vi "ttl_high_low.vi"(4 "lines":tag="Dev1/port2/line7", 7 "Boolean":bool=TRUE) -> ()   [LabVIEW 2011]
uses:
  <vilib>/DAQmx/write.llb/DAQmx Write (Digital 1D Bool 1Chan 1Samp).vi
  <vilib>/DAQmx/create/channels.llb/DAQmx Create Channel (DO-Digital Output).vi
  <vilib>/DAQmx/miscellaneous.llb/DAQmx Fill In Error Info.vi
  Program Files/National Instruments/LabVIEW 2011/resource/objmgr/daqmx.rc
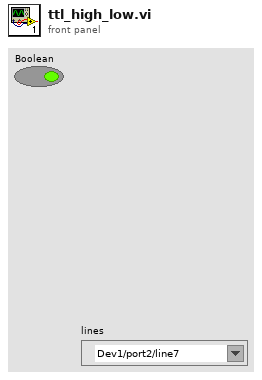
[diagram p1: front panel]
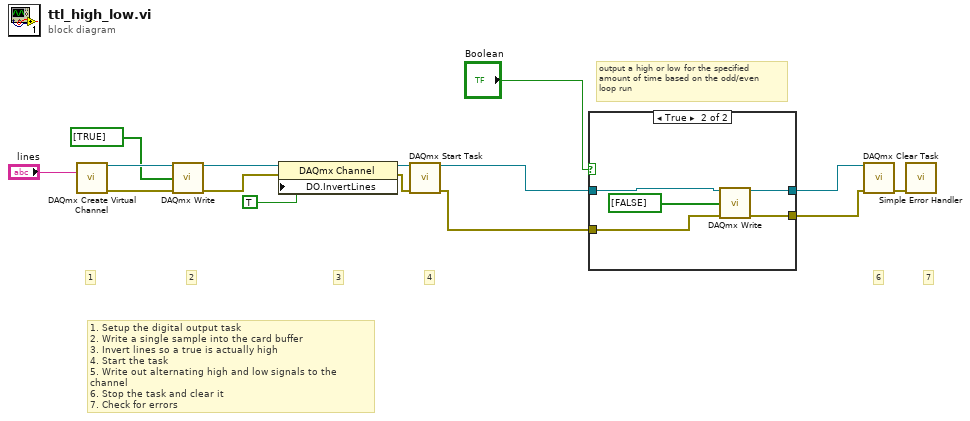
[diagram p0: block diagram]
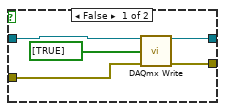
[diagram p2: hidden frame]
diagram:
  # "output a high or low for the specified\namount of time based on the odd/even\nloop run"
  # "1. Setup the digital output task\n2. Write a single sample into the card buffer\n3. Invert lines so a true is actually high\n4. Start the task\n5. Write out alternating high and low signals to the channel\n6. Stop the task and clear it\n7. Check for errors"
  # "7"
  # "6"
  # "4"
  # "3"
  # "2"
  # "1"
  n1 = call-poly <vilib>:"DAQmx Create Virtual Channel.vi"("lines"="lines") -> ("task out"=w15:refnum<k21>, "error out"=w14:errorcluster)  [unwired: 13 in]
  n2 = call-poly <vilib>:"DAQmx Write.vi"("task/channels in"=w15, "data"=bool[] [TRUE], "error in"=w14) -> ("task out"=w10:refnum<k21>, "error out"=w6:errorcluster)  [unwired: 10 in, 1 out]
  n3 = property class="DAQmx Channel"(reference=w10, error in=w6, "DO.InvertLines"=TRUE) -> (reference out=w9:refnum<k21>, error out=w8:errorcluster)
  n4 = call <vilib>:"DAQmx Start Task.vi"("task/channels in"=w9, "error in"=w8) -> ("task out"=w4:refnum<k21>, "error out"=w3:errorcluster)  [unwired: 12 in]
  n5 = case shown="True" "Boolean" {
    tunnel: [w19 w25] -> w1
    tunnel: [w18 w24] -> w2
    tunnel: w4 -> [w16 w21]
    tunnel: w3 -> [w17 w22]
    frame False {
      n6 = call-poly <vilib>:"DAQmx Write.vi"("task/channels in"=w16, "data"=bool[] [TRUE], "error in"=w17) -> ("task out"=w18:refnum<k21>, "error out"=w19:errorcluster)  [unwired: 10 in, 1 out]
    }
    frame True {
      n7 = call-poly <vilib>:"DAQmx Write.vi"("task/channels in"=w21, "data"=bool[] [FALSE], "error in"=w22) -> ("task out"=w24:refnum<k21>, "error out"=w25:errorcluster)  [unwired: 10 in, 1 out]
    }
  }
  n8 = call <vilib>:"DAQmx Clear Task.vi"("task in"=w2, "error in"=w1) -> ("error out"=w13:errorcluster)  [unwired: 13 in]
  n9 = call <vilib>:"Simple Error Handler.vi"("error in (no error)"=w13) -> ()  [unwired: 4 in, 5 out]
